vi "Time series viewer-Event handler-Exit.vi"(11 "Queue in":refnum<queue>) -> (2 "Exit":bool)   [LabVIEW 2020]
uses:
  Typedefs/Speed Viewer States enum.ctl
  Globals/gl_Time series viewer globals.vi
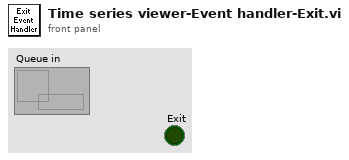
[diagram p1: front panel]
types:
  T1 = typedef "Time series viewer refs.ctl" = cluster{"This VI":refnum<vi>, "Image control":refnum<vi>, "AVI Mode ind":refnum<vi>, "Play":refnum<vi>, "Stop":refnum<vi>, "Back":refnum<vi>, "Scrollbar":refnum<vi>, "Video length info":refnum<vi>, "Expected speed values":refnum<vi>, "Intensity":refnum<vi>, "Path":refnum<vi>, "Selection sliders":refnum<vi>, "Speed Graph ref":refnum<vi>, "Frame rate set (fps)":refnum<vi>, "Number of rows to generate":refnum<vi>, "VL Image Array":refnum<vi>, "Image Scrollbar":refnum<vi>, "Channel to load":refnum<vi>, "Colour":refnum<vi>}
  T2 = typedef "Speed Viewer States enum.ctl" = enum16{"Idle", "Initialise", "Playback", "Scroll bar event", "Speed cursor event", "Back to start", "Exit"}
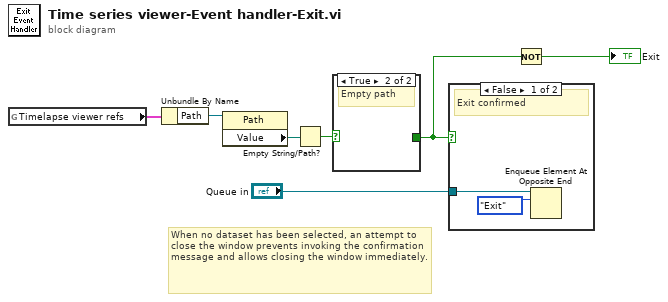
[diagram p0: block diagram]
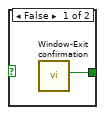
[diagram p2: hidden frame]
diagram:
  # "When no dataset has been selected, an attempt to close the window prevents invoking the confirmation message and allows closing the window immediately."
  n1 = global read "gl_Time series viewer globals.vi" "Timelapse viewer refs"() -> (w4:T1)
  n2 = Unbundle By Name(w4) -> ("Path"=w3:refnum<vi>)
  n3 = property class="Path"(reference=w3) -> ("Value"=w2:path)  [unwired: 1 in, 2 out]
  n4 = Empty String/Path?(string/path=w2) -> (empty?=w1:bool)
  n5 = case shown="True" w1 {
    tunnel: [w8 _] -> w6
    frame False {
      n6 = call "Window-Exit confirmation.vi"() -> ("Cancelled"=w8:bool)  [unwired: 10 in, 1 out]
    }
    frame True {
      # "Empty path"
    }
  }
  n7 = case shown="False" w6 {
    tunnel: "Queue in" -> [w9 _]
    frame False {
      # "Exit confirmed"
      n8 = Enqueue Element At Opposite End(queue=w9, element=Speed_Viewer_States_enum."Exit" ("States")) -> ()  [unwired: 2 in, 3 out]
    }
    frame True {
      # "Cancelled"
    }
  }
  n9 = Not(x=w6) -> (.not. x?=→"Exit":bool)
